vi "Main.vi"() -> ()   [LabVIEW 2020]
uses:
  DVR-Module/DVR-Module.lvlib
panel:
  out "dbl 6":dbl
  out "dbl 5":dbl
  out "dbl 4":dbl
  out "dbl 3":dbl
  out "dbl 2":dbl
  out "dbl":dbl
  # "dvr module"
  # "fgv module"
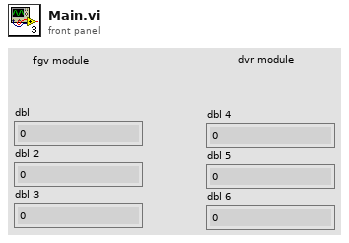
[diagram p1: front panel]
types:
  T1 = enum16{"Initialize", "Random", "Read", "Write", "Close"}
  T2 = typedef "DVR-Module.lvlib/DVR.ctl" = refnum<data-value>
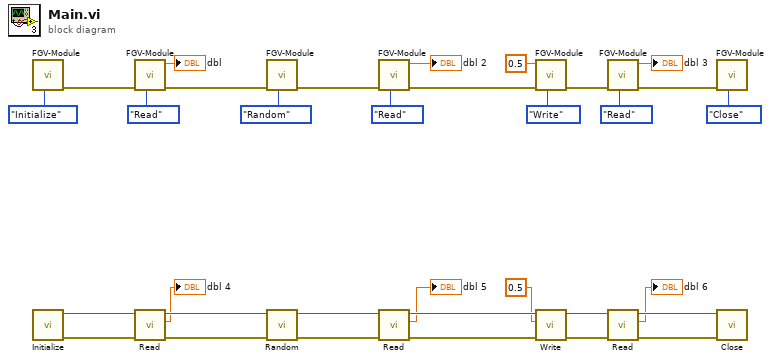
[diagram p0: block diagram]
diagram:
  n1 = call "FGV-Module.vi"("Operation"=T1."Initialize") -> ("Error out"=w31:errorcluster)  [unwired: 9 in, 1 out]
  n2 = call "Initialize.vi"() -> ("error out"=w15:errorcluster, "DVR"=w16:T2)  [unwired: 10 in]
  n3 = call "FGV-Module.vi"("Operation"=T1."Read", "Error in"=w31) -> ("Error out"=w29:errorcluster, "dbl"=→"dbl":dbl)  [unwired: 8 in]
  n4 = call "Read.vi"("Error in"=w15, "DVR"=w16) -> ("Error out"=w13:errorcluster, "dbl"=→"dbl 4":dbl, "DVR(dup)"=w14:T2)  [unwired: 7 in]
  n5 = call "FGV-Module.vi"("Operation"=T1."Random", "Error in"=w29) -> ("Error out"=w27:errorcluster)  [unwired: 8 in, 1 out]
  n6 = call "Random.vi"("Error in"=w13, "DVR"=w14) -> ("Error out"=w11:errorcluster, "DVR(dup)"=w12:T2)  [unwired: 8 in]
  n7 = call "FGV-Module.vi"("Operation"=T1."Read", "Error in"=w27) -> ("Error out"=w25:errorcluster, "dbl"=→"dbl 2":dbl)  [unwired: 8 in]
  n8 = call "Read.vi"("Error in"=w11, "DVR"=w12) -> ("Error out"=w9:errorcluster, "dbl"=→"dbl 5":dbl, "DVR(dup)"=w10:T2)  [unwired: 7 in]
  n9 = call "FGV-Module.vi"("Operation"=T1."Write", "Error in"=w25, "input"=0.5) -> ("Error out"=w23:errorcluster)  [unwired: 7 in, 1 out]
  n10 = call "Write.vi"("Error in"=w9, "dbl"=0.5 ("input"), "DVR"=w10) -> ("Error out"=w7:errorcluster, "DVR(dup)"=w8:T2)  [unwired: 7 in]
  n11 = call "FGV-Module.vi"("Operation"=T1."Read", "Error in"=w23) -> ("Error out"=w21:errorcluster, "dbl"=→"dbl 3":dbl)  [unwired: 8 in]
  n12 = call "Read.vi"("Error in"=w7, "DVR"=w8) -> ("Error out"=w5:errorcluster, "dbl"=→"dbl 6":dbl, "DVR(dup)"=w6:T2)  [unwired: 7 in]
  n13 = call "FGV-Module.vi"("Operation"=T1."Close", "Error in"=w21) -> ()  [unwired: 8 in, 2 out]
  n14 = call "Close.vi"("Error in"=w5, "DVR"=w6) -> ()  [unwired: 8 in, 2 out]
